vi "TopLevel.vi"() -> ()   [LabVIEW 2020]
panel:
  out "Turn within threshold?":bool
  in  "Good Turn Threshold":dbl=0.1
  in  "Turn Gains":T1
  in  "Desired Heading":dbl=5.0
  out "Car Position":cluster{"X":dbl, "Y":dbl}[](graph)
  out "Speed within threshold?":bool
  in  "Good Speed Threshold":dbl=0.1
  in  "Speed Gains":T1={"kP"=1.0, "kI"=0.01, "kD"=1.0, "iZone"=1.0}
  out "output":dbl format="%.2f"
  out "PhysicalProperties":T2(graph)
  in  "Desired Speed":dbl=5.0
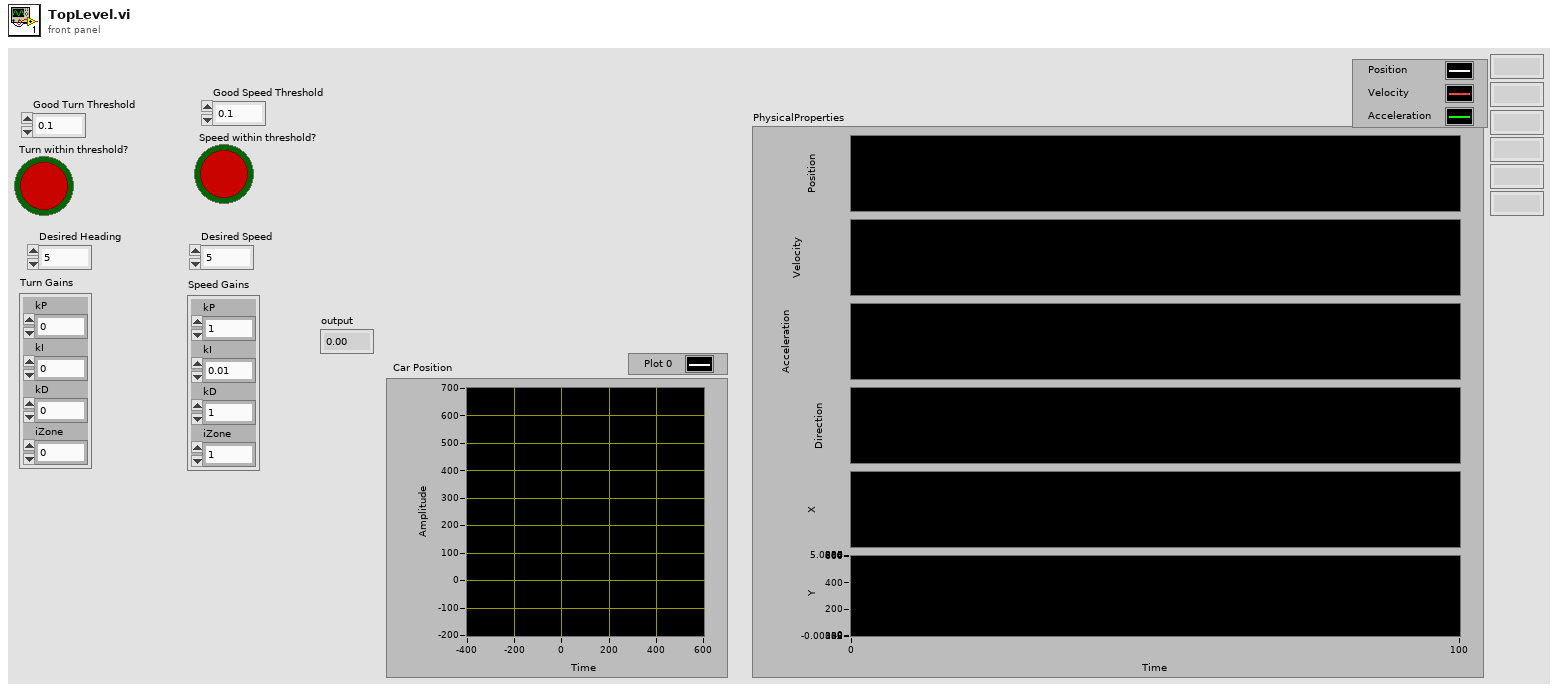
[diagram p1: front panel]
types:
  T1 = cluster{"kP":dbl, "kI":dbl, "kD":dbl, "iZone":dbl}
  T2 = cluster{"Position":dbl, "Velocity":dbl, "Acceleration":dbl, "Direction":dbl, "X":dbl, "Y":dbl}
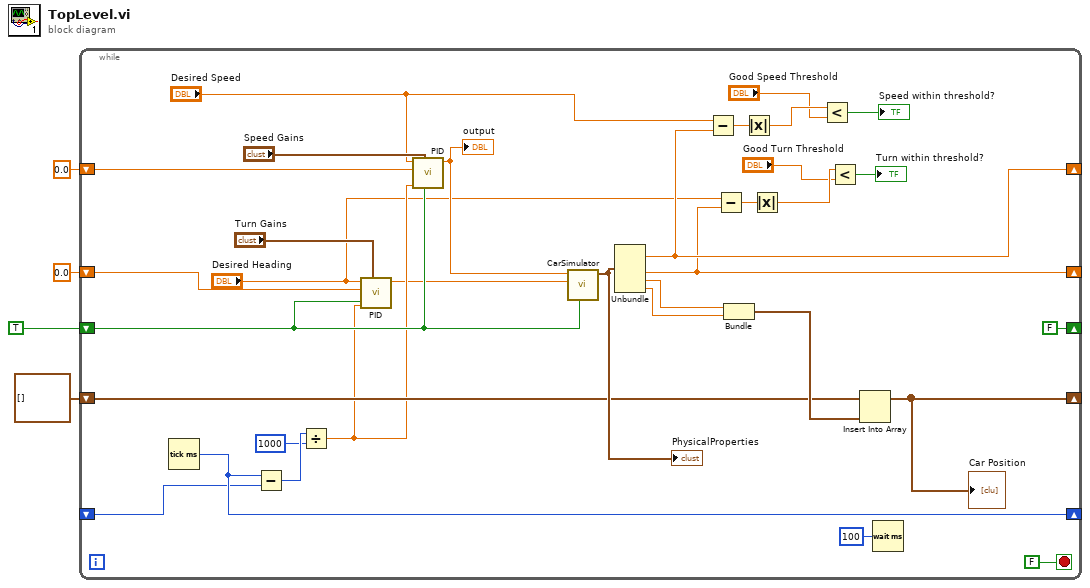
[diagram p0: block diagram]
diagram:
  n1 = while {
    shift-right: [w22] -> _
    shift-left: 0.0 ("Velocity") -> [w30]
    shift-right: [w35] -> _
    shift-left: _ -> [w34]
    shift-right: [FALSE] -> _
    shift-left: TRUE -> [w15]
    shift-right: [w17] -> _
    shift-left: cluster{"X":dbl, "Y":dbl}[] [] -> [w16]
    shift-right: [w6] -> _
    shift-left: 0.0 ("Direction") -> [w11]
    stop <- FALSE stop-if-true
    n2 = Tick Count (ms)() -> (millisecond timer value=w35:u32)
    n3 = Subtract(x=w35, y=w34) -> (x-y=w33:u32)
    n4 = Divide(x=w33, y=u32 1000) -> (x/y=w14:dbl)
    n5 = call "PID.vi"("Reinit"=w15, "Gains"="Turn Gains", "dT"=w14, "Current"=w11, "Target"="Desired Heading") -> ("Out"=w13:dbl)  [unwired: 6 in]
    n6 = call "PID.vi"("Reinit"=w15, "Gains"="Speed Gains", "dT"=w14, "Current"=w30, "Target"="Desired Speed") -> ("Out"=w29:dbl)  [unwired: 6 in]
    "output" <- w29
    n7 = call "CarSimulator.vi"("Reinit"=w15, "Steering Control"=w13, "Brake/Gas Control"=w29) -> ("PhysicalProperties"=w21:T2)  [unwired: 8 in]
    "PhysicalProperties" <- w21
    n8 = Unbundle(w21) -> ("Velocity"=w22:dbl, "Direction"=w6:dbl, "X"=w20:dbl, "Y"=w19:dbl)  [unwired: 2 out]
    n9 = Subtract(x="Desired Speed", y=w22) -> (x-y=w26:dbl)
    n10 = Subtract(x="Desired Heading", y=w6) -> (x-y=w10:dbl)
    n11 = Bundle("X"=w20, "Y"=w19) -> (w18:cluster{"X":dbl, "Y":dbl})  [unwired: 1 in]
    n12 = Absolute Value(x=w26) -> (abs(x)=w25:dbl)
    n13 = Absolute Value(x=w10) -> (abs(x)=w9:dbl)
    n14 = Less?(x=w25, y="Good Speed Threshold") -> (x < y?=→"Speed within threshold?":bool)
    n15 = Less?(x=w9, y="Good Turn Threshold") -> (x < y?=→"Turn within threshold?":bool)
    n16 = Insert Into Array(array=w16, new element=w18) -> (w17:cluster{"X":dbl, "Y":dbl}[])  [unwired: 1 in]
    "Car Position" <- w17
    n17 = Wait (ms)(milliseconds to wait=u32 100) -> ()  [unwired: 1 out]
  }
